vi "Open Instrument.vi"(8 "error in (no error)":errorcluster, 11 "instrument.Cryostation in":refnum<class "instrument.Cryostation.lvclass">) -> (0 "error out":errorcluster, 3 "instrument.Cryostation out":refnum<class "instrument.Cryostation.lvclass">)   [LabVIEW 2016, in "instrument.Cryostation.lvclass"]
uses:
  instrument.Cryostation.lvclass
  instrument.Cryostation.lvclass/instrument.Cryostation.ctl
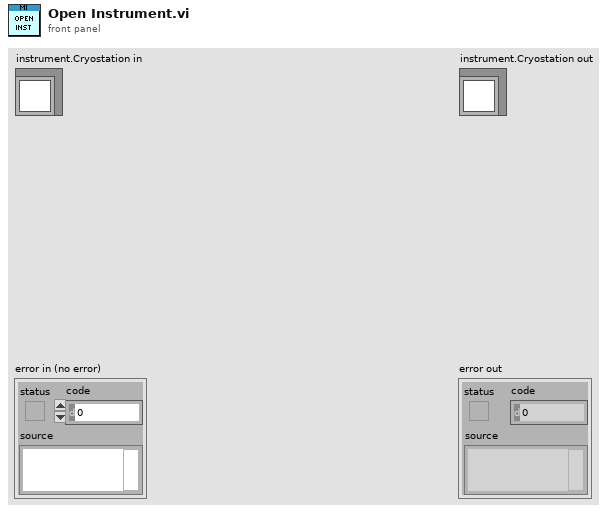
[diagram p1: front panel]
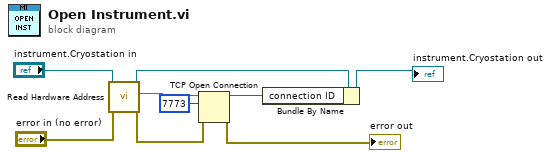
[diagram p0: block diagram]
diagram:
  n1 = call-dynamic "Read Hardware Address.vi"("error in (no error)"="error in (no error)", "Instrument in"="instrument.Cryostation in") -> ("error out"=w4:errorcluster, "Hardware Address"=w8:string, "Instrument out"=w1:refnum<class "instrument.Cryostation.lvclass">)  [unwired: 7 in]
  n2 = TCP Open Connection(address=w8, remote port or service name=u16 7773, error in (no error)=w4) -> (connection ID=w3:refnum<k5>, error out=→"error out":errorcluster)  [unwired: 2 in]
  n3 = Bundle By Name(cluster=w1, "connection ID"=w3) -> (→"instrument.Cryostation out":refnum<class "instrument.Cryostation.lvclass">)
